vi "Autonomous Independent.vi"   [LabVIEW 2017]
doc: "This VI is called when autonomous begins, and will automatically be terminated when autonomous ends. You can carry out timed or sensor driven robot movement independently without needing to return to the caller."
uses:
  <vilib>/Rock Robotics/WPI/Utilities/WPI_GetSetVariantRefNum.vi
  <vilib>/Rock Robotics/Network Tables/NT Read String.vi
  <vilib>/Rock Robotics/Network Tables/NT Write Numeric Array.vi
  <vilib>/Rock Robotics/Network Tables/NT Read Number.vi
panel:
  # "Be sure to right-click and choose Data Operations>>Make Current Value default if you want to save the array values with the VI"
types:
  T1 = typedef "WPI_JoystickDevRef.ctl" = cluster{"Device":T2}
  T2 = typedef "WPI_JoystickDeviceEnum.ctl" = enum16{"USB 0", "USB 1", "USB 2", "USB 3", "USB 4", "USB 5"}
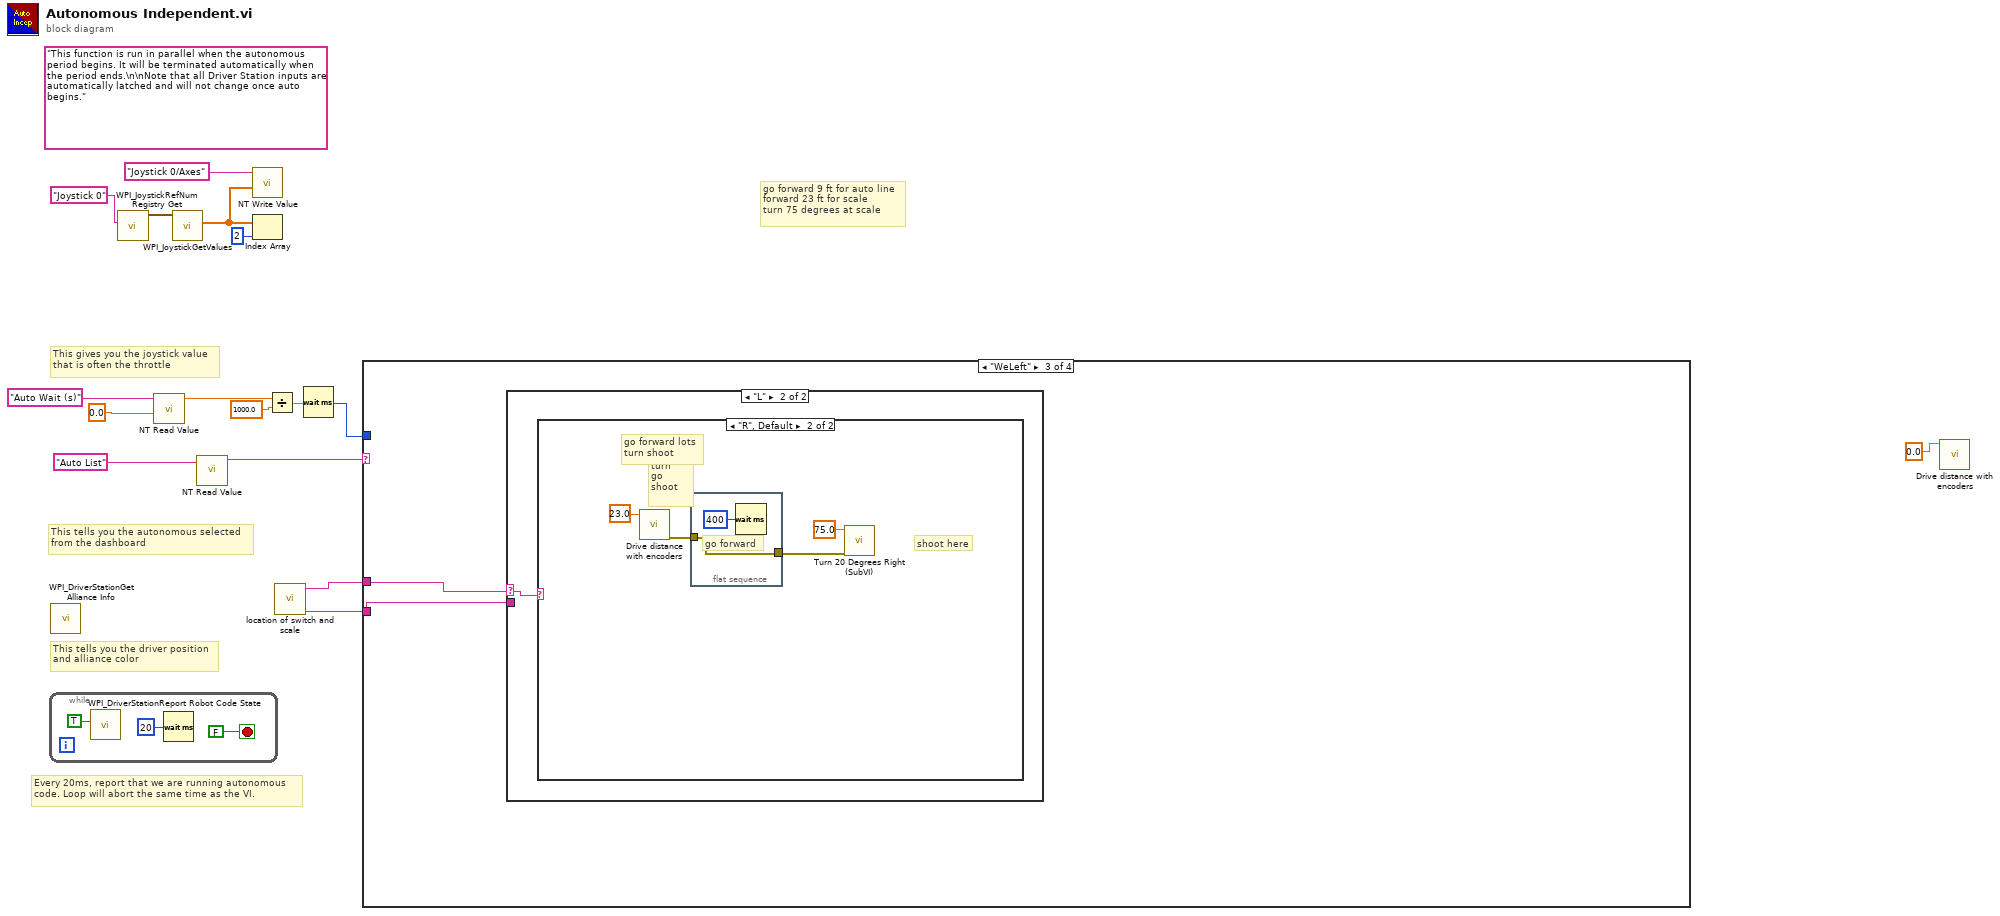
[diagram p0: block diagram]
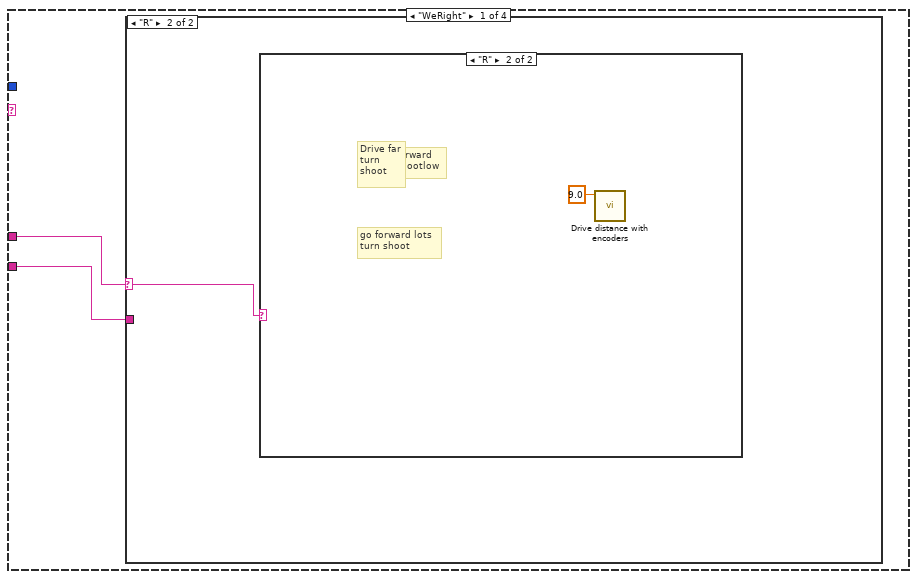
[diagram p2: hidden frame]
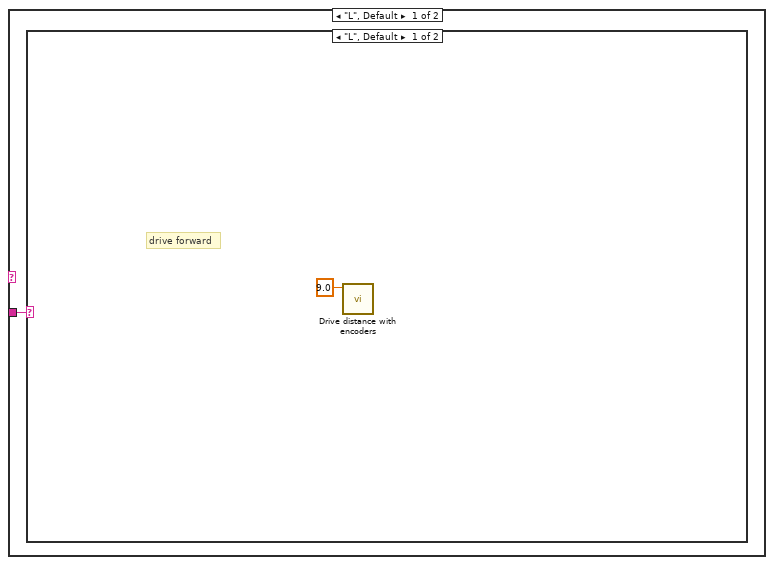
[diagram p3: hidden frame]
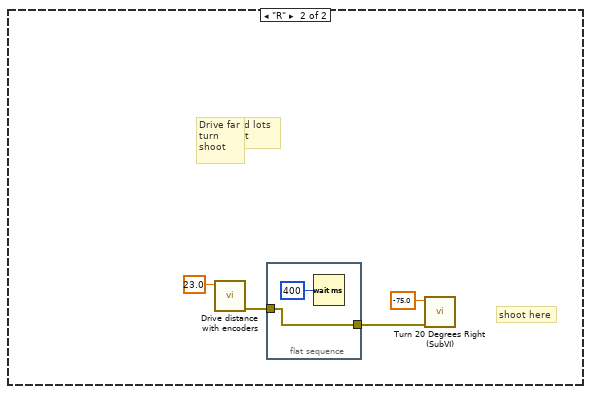
[diagram p4: hidden frame]
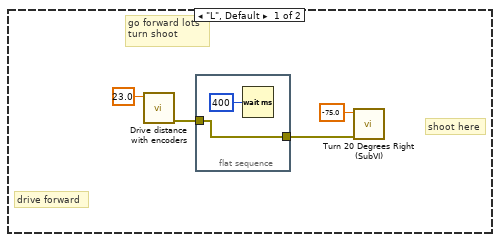
[diagram p5: hidden frame]
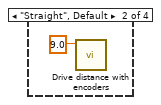
[diagram p6: hidden frame]
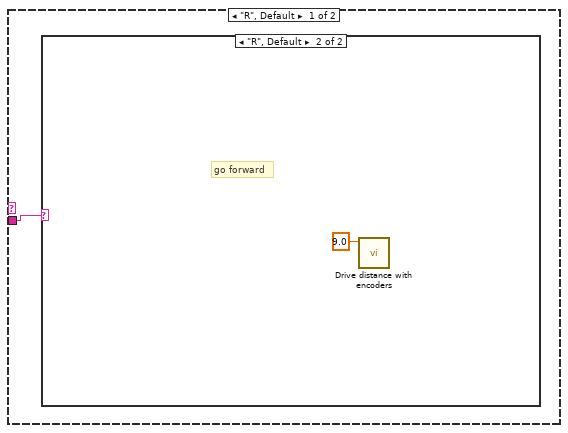
[diagram p7: hidden frame]
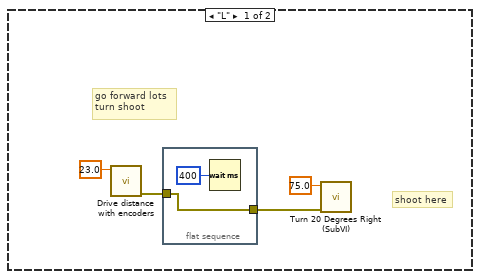
[diagram p8: hidden frame]
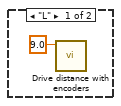
[diagram p9: hidden frame]
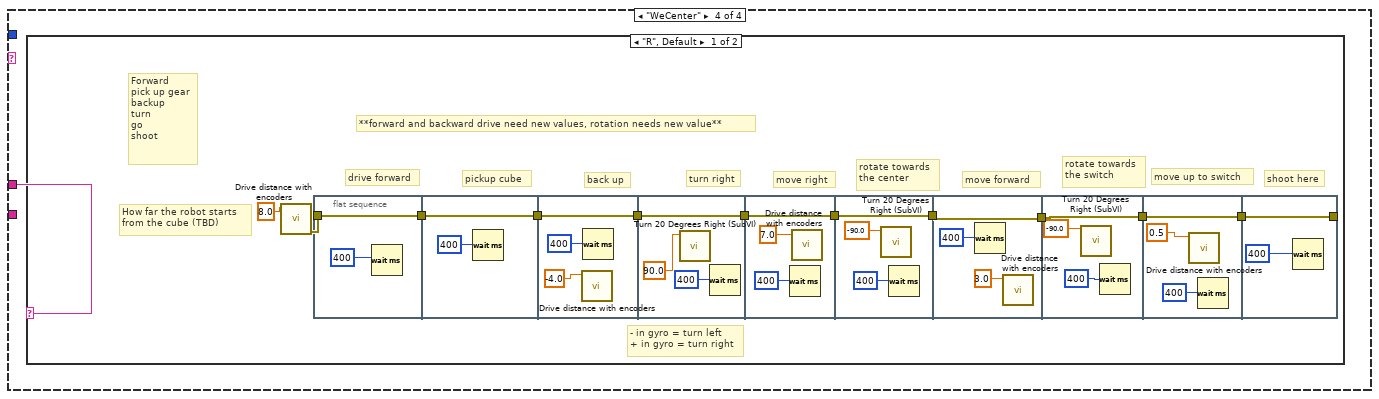
[diagram p10: hidden frame]
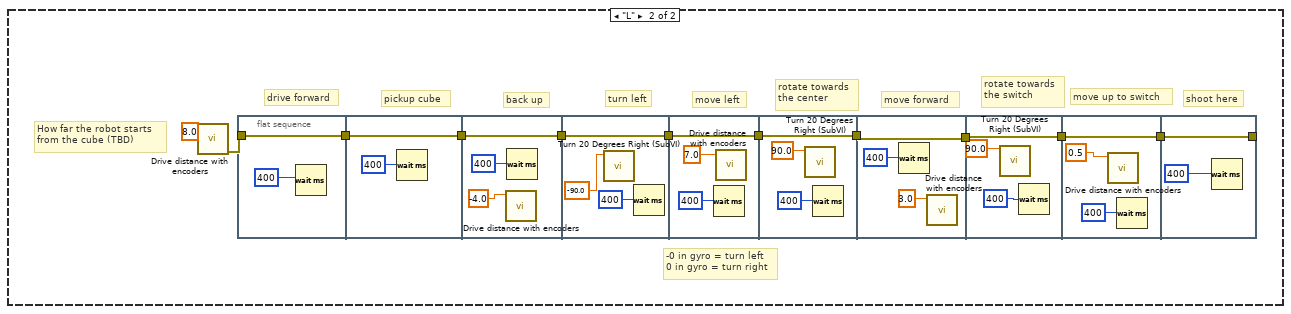
[diagram p11: hidden frame]
diagram:
  (unwired) "This function is run in parallel when the autonomous period begins. It will be terminated automatically when the period ends.\n\nNote that all Driver Station inputs are automatically latched and will not change once auto begins."
  # "go forward 9 ft for auto line\nforward 23 ft for scale\nturn 75 degrees at scale"
  # "This tells you the autonomous selected\nfrom the dashboard"
  # "Every 20ms, report that we are running autonomous\ncode. Loop will abort the same time as the VI."
  # "This gives you the joystick value\nthat is often the throttle"
  # "This tells you the driver position\nand alliance color"
  n1 = while {
    stop <- FALSE stop-if-true
    n2 = call <vilib>:"WPI_DriverStationReport Robot Code State.vi"("Autonomous"=TRUE) -> ()  [unwired: 10 in, 1 out]
    n3 = Wait (ms)(milliseconds to wait=u32 20) -> ()  [unwired: 1 out]
  }
  n4 = call <vilib>:"WPI_DriverStationGet Alliance Info.vi"() -> ()  [unwired: 12 out]
  n5 = call <vilib>:"WPI_JoystickRefNum Registry Get.vi"("refnum name"="Joystick 0") -> ("JoystickDevRef"=w15:T1)  [unwired: 1 in, 9 out]
  n6 = call-poly <vilib>:"NT Read Value.vi"("Default Value"=0.0, "Name"="Auto Wait (s)") -> ("Numeric"=w4:dbl)  [unwired: 8 in, 1 out]
  n7 = call <vilib>:"WPI_JoystickGetValues.vi"("JoystickDevRef"=w15) -> ("Axes"=w11:dbl[])  [unwired: 6 in, 4 out]
  n8 = call-poly <vilib>:"NT Read Value.vi"("Name"="Auto List") -> ("String"=w12:string)  [unwired: 9 in, 1 out]
  n9 = call-poly <vilib>:"NT Write Value.vi"("Numeric Array"=w11, "Name"="Joystick 0/Axes") -> ()  [unwired: 9 in, 1 out]
  n10 = Index Array(array=w11, index=2) -> ()  [unwired: 1 out]
  n11 = Divide(x=w4, y=1000.0) -> (x/y=w3:dbl)
  n12 = call "location of switch and scale.vi"() -> ("Scale"=w8:string, "Switch"=w9:string)  [unwired: 10 in]
  n13 = Wait (ms)(milliseconds to wait=w3) -> (millisecond timer value=w7:u32)
  n14 = case shown="\"WeLeft\"" w12 {
    tunnel: w9 -> [w21 _ w40 w57]
    tunnel: w8 -> [w20 _ w39 _]
    tunnel: w7 -> [_ _ _ _]
    frame "WeRight" {
      n15 = case shown="\"R\"" w21 {
        selector: w21 -> [_ w30]
        tunnel: w20 -> [w22 _]
        frame "L", Default {
          n16 = case shown="\"L\", Default" w22 {
            frame "L", Default {
              # "drive forward"
              n17 = call "Drive distance with encoders.vi"("Wanted Distance"=9.0) -> ()  [unwired: 10 in, 1 out]
            }
            frame "R" {
              # "shoot here"
              # "go forward lots\nturn shoot"
              # "Drive far\nturn\nshoot"
              n18 = call "Drive distance with encoders.vi"("Wanted Distance"=23.0) -> ("error out"=w26:errorcluster)  [unwired: 10 in]
              n19 = flat-sequence {
                tunnel: w26 -> [w28]
                tunnel: [w28] -> w25
                frame #0 {
                  n20 = Wait (ms)(milliseconds to wait=u32 400) -> ()  [unwired: 1 out]
                }
              }
              n21 = call "Turn 20 Degrees Right (SubVI).vi"("error in (no error)"=w25, "Turn? Right Positive."=-75.0) -> ()  [unwired: 9 in, 1 out]
            }
          }
        }
        frame "R" {
          # "forward\nshootlow"
          n22 = case shown="\"R\"" w30 {
            frame "L", Default {
              # "shoot here"
              # "go forward lots\nturn shoot"
              # "drive forward"
              n23 = call "Drive distance with encoders.vi"("Wanted Distance"=23.0) -> ("error out"=w33:errorcluster)  [unwired: 10 in]
              n24 = flat-sequence {
                tunnel: w33 -> [w35]
                tunnel: [w35] -> w34
                frame #0 {
                  n25 = Wait (ms)(milliseconds to wait=u32 400) -> ()  [unwired: 1 out]
                }
              }
              n26 = call "Turn 20 Degrees Right (SubVI).vi"("error in (no error)"=w34, "Turn? Right Positive."=-75.0) -> ()  [unwired: 9 in, 1 out]
            }
            frame "R" {
              # "go forward lots\nturn shoot"
              # "Drive far\nturn\nshoot"
              n27 = call "Drive distance with encoders.vi"("Wanted Distance"=9.0) -> ()  [unwired: 10 in, 1 out]
            }
          }
        }
      }
    }
    frame "Straight", Default {
      n28 = call "Drive distance with encoders.vi"("Wanted Distance"=9.0) -> ()  [unwired: 10 in, 1 out]
    }
    frame "WeLeft" {
      n29 = case shown="\"L\"" w40 {
        selector: w40 -> [_ w49]
        tunnel: w39 -> [w41 _]
        frame "R", Default {
          n30 = case shown="\"R\", Default" w41 {
            frame "L" {
              # "shoot here"
              # "go forward lots\nturn shoot"
              n31 = call "Drive distance with encoders.vi"("Wanted Distance"=23.0) -> ("error out"=w44:errorcluster)  [unwired: 10 in]
              n32 = flat-sequence {
                tunnel: w44 -> [w46]
                tunnel: [w46] -> w43
                frame #0 {
                  n33 = Wait (ms)(milliseconds to wait=u32 400) -> ()  [unwired: 1 out]
                }
              }
              n34 = call "Turn 20 Degrees Right (SubVI).vi"("error in (no error)"=w43, "Turn? Right Positive."=75.0) -> ()  [unwired: 9 in, 1 out]
            }
            frame "R", Default {
              # "go forward"
              n35 = call "Drive distance with encoders.vi"("Wanted Distance"=9.0) -> ()  [unwired: 10 in, 1 out]
            }
          }
        }
        frame "L" {
          # "Forward\nturn\ngo\nshoot"
          n36 = case shown="\"R\", Default" w49 {
            frame "L" {
              n37 = call "Drive distance with encoders.vi"("Wanted Distance"=9.0) -> ()  [unwired: 10 in, 1 out]
            }
            frame "R", Default {
              # "shoot here"
              # "go forward lots\nturn shoot"
              # "go forward"
              n38 = call "Drive distance with encoders.vi"("Wanted Distance"=23.0) -> ("error out"=w53:errorcluster)  [unwired: 10 in]
              n39 = flat-sequence {
                tunnel: w53 -> [w55]
                tunnel: [w55] -> w52
                frame #0 {
                  n40 = Wait (ms)(milliseconds to wait=u32 400) -> ()  [unwired: 1 out]
                }
              }
              n41 = call "Turn 20 Degrees Right (SubVI).vi"("error in (no error)"=w52, "Turn? Right Positive."=75.0) -> ()  [unwired: 9 in, 1 out]
            }
          }
        }
      }
    }
    frame "WeCenter" {
      n42 = case shown="\"R\", Default" w57 {
        frame "R", Default {
          # "- in gyro = turn left\n+ in gyro = turn right"
          # "shoot here"
          # "move up to switch"
          # "rotate towards \nthe switch"
          # "move forward"
          # "rotate towards \nthe center"
          # "move right"
          # "**forward and backward drive need new values, rotation needs new value**"
          # "turn right"
          # "back up"
          # "drive forward"
          # "pickup cube"
          # "How far the robot starts \nfrom the cube (TBD)"
          # "Forward\npick up gear\nbackup\nturn\ngo\nshoot"
          n43 = call "Drive distance with encoders.vi"("Wanted Distance"=8.0) -> ("error out"=w58:errorcluster)  [unwired: 10 in]
          n44 = flat-sequence {
            tunnel: w58 -> [w70]
            tunnel: [w70] -> w59
            tunnel: [w72] -> w60
            tunnel: w59 -> [w72]
            tunnel: [w75] -> w61
            tunnel: w60 -> [w75]
            tunnel: [w78] -> w62
            tunnel: w61 -> [w78]
            tunnel: [w81] -> w63
            tunnel: w62 -> [w81]
            tunnel: [w84] -> w64
            tunnel: w63 -> [w84]
            tunnel: [w87] -> w65
            tunnel: w64 -> [w87]
            tunnel: [w89] -> w67
            tunnel: w65 -> [w89]
            tunnel: w67 -> [w93]
            tunnel: [w93] -> w66
            tunnel: [w95] -> _
            tunnel: w66 -> [w95]
            frame #0 {
              n45 = Wait (ms)(milliseconds to wait=u32 400) -> ()  [unwired: 1 out]
            }
            frame #1 {
              n46 = Wait (ms)(milliseconds to wait=u32 400) -> ()  [unwired: 1 out]
            }
            frame #2 {
              n47 = call "Drive distance with encoders.vi"("Wanted Distance"=-4.0) -> ()  [unwired: 10 in, 1 out]
              n48 = Wait (ms)(milliseconds to wait=u32 400) -> ()  [unwired: 1 out]
            }
            frame #3 {
              n49 = call "Turn 20 Degrees Right (SubVI).vi"("Turn? Right Positive."=90.0) -> ()  [unwired: 10 in, 1 out]
              n50 = Wait (ms)(milliseconds to wait=u32 400) -> ()  [unwired: 1 out]
            }
            frame #4 {
              n51 = Wait (ms)(milliseconds to wait=u32 400) -> ()  [unwired: 1 out]
              n52 = call "Drive distance with encoders.vi"("Wanted Distance"=7.0) -> ()  [unwired: 10 in, 1 out]
            }
            frame #5 {
              n53 = call "Turn 20 Degrees Right (SubVI).vi"("Turn? Right Positive."=-90.0) -> ()  [unwired: 10 in, 1 out]
              n54 = Wait (ms)(milliseconds to wait=u32 400) -> ()  [unwired: 1 out]
            }
            frame #6 {
              n55 = Wait (ms)(milliseconds to wait=u32 400) -> ()  [unwired: 1 out]
              n56 = call "Drive distance with encoders.vi"("Wanted Distance"=3.0) -> ()  [unwired: 10 in, 1 out]
            }
            frame #7 {
              n57 = call "Turn 20 Degrees Right (SubVI).vi"("Turn? Right Positive."=-90.0) -> ()  [unwired: 10 in, 1 out]
              n58 = Wait (ms)(milliseconds to wait=u32 400) -> ()  [unwired: 1 out]
            }
            frame #8 {
              n59 = call "Drive distance with encoders.vi"("Wanted Distance"=0.5) -> ()  [unwired: 10 in, 1 out]
              n60 = Wait (ms)(milliseconds to wait=u32 400) -> ()  [unwired: 1 out]
            }
            frame #9 {
              n61 = Wait (ms)(milliseconds to wait=u32 400) -> ()  [unwired: 1 out]
            }
          }
        }
        frame "L" {
          # "-0 in gyro = turn left\n0 in gyro = turn right"
          # "shoot here"
          # "move up to switch"
          # "rotate towards \nthe switch"
          # "move forward"
          # "rotate towards \nthe center"
          # "move left"
          # "turn left"
          # "back up"
          # "drive forward"
          # "pickup cube"
          # "How far the robot starts \nfrom the cube (TBD)"
          n62 = call "Drive distance with encoders.vi"("Wanted Distance"=8.0) -> ("error out"=w96:errorcluster)  [unwired: 10 in]
          n63 = flat-sequence {
            tunnel: w96 -> [w108]
            tunnel: [w108] -> w106
            tunnel: [w110] -> w105
            tunnel: w106 -> [w110]
            tunnel: [w113] -> w104
            tunnel: w105 -> [w113]
            tunnel: [w116] -> w103
            tunnel: w104 -> [w116]
            tunnel: [w119] -> w102
            tunnel: w103 -> [w119]
            tunnel: [w122] -> w101
            tunnel: w102 -> [w122]
            tunnel: [w125] -> w100
            tunnel: w101 -> [w125]
            tunnel: [w127] -> w99
            tunnel: w100 -> [w127]
            tunnel: w99 -> [w131]
            tunnel: [w131] -> w98
            tunnel: [w133] -> _
            tunnel: w98 -> [w133]
            frame #0 {
              n64 = Wait (ms)(milliseconds to wait=u32 400) -> ()  [unwired: 1 out]
            }
            frame #1 {
              n65 = Wait (ms)(milliseconds to wait=u32 400) -> ()  [unwired: 1 out]
            }
            frame #2 {
              n66 = call "Drive distance with encoders.vi"("Wanted Distance"=-4.0) -> ()  [unwired: 10 in, 1 out]
              n67 = Wait (ms)(milliseconds to wait=u32 400) -> ()  [unwired: 1 out]
            }
            frame #3 {
              n68 = call "Turn 20 Degrees Right (SubVI).vi"("Turn? Right Positive."=-90.0) -> ()  [unwired: 10 in, 1 out]
              n69 = Wait (ms)(milliseconds to wait=u32 400) -> ()  [unwired: 1 out]
            }
            frame #4 {
              n70 = Wait (ms)(milliseconds to wait=u32 400) -> ()  [unwired: 1 out]
              n71 = call "Drive distance with encoders.vi"("Wanted Distance"=7.0) -> ()  [unwired: 10 in, 1 out]
            }
            frame #5 {
              n72 = call "Turn 20 Degrees Right (SubVI).vi"("Turn? Right Positive."=90.0) -> ()  [unwired: 10 in, 1 out]
              n73 = Wait (ms)(milliseconds to wait=u32 400) -> ()  [unwired: 1 out]
            }
            frame #6 {
              n74 = Wait (ms)(milliseconds to wait=u32 400) -> ()  [unwired: 1 out]
              n75 = call "Drive distance with encoders.vi"("Wanted Distance"=3.0) -> ()  [unwired: 10 in, 1 out]
            }
            frame #7 {
              n76 = call "Turn 20 Degrees Right (SubVI).vi"("Turn? Right Positive."=90.0) -> ()  [unwired: 10 in, 1 out]
              n77 = Wait (ms)(milliseconds to wait=u32 400) -> ()  [unwired: 1 out]
            }
            frame #8 {
              n78 = call "Drive distance with encoders.vi"("Wanted Distance"=0.5) -> ()  [unwired: 10 in, 1 out]
              n79 = Wait (ms)(milliseconds to wait=u32 400) -> ()  [unwired: 1 out]
            }
            frame #9 {
              n80 = Wait (ms)(milliseconds to wait=u32 400) -> ()  [unwired: 1 out]
            }
          }
        }
      }
    }
  }
  n81 = call "Drive distance with encoders.vi"("Wanted Distance"=0.0) -> ()  [unwired: 10 in, 1 out]
